vi "Try Parse.vi"(0 "Path Group in":refnum<class "Path Group.lvclass">, 5 "Config Rows":string[][](array[string]), 11 "error in (no error)":errorcluster) -> (4 "Path Group out":refnum<class "Path Group.lvclass">, 6 "Unparsed Rows":string[][](array[string]), 10 "Path Count":i32, 15 "error out":errorcluster)   [LabVIEW 2023, in "RFCalAndFixtureCharact.Common.lvlib" / "Path Group.lvclass"]
uses:
  Path Group.lvclass
  Path/Path.lvclass
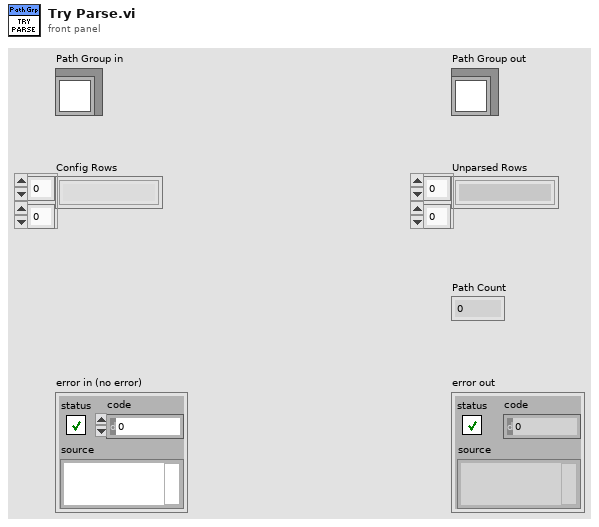
[diagram p1: front panel]
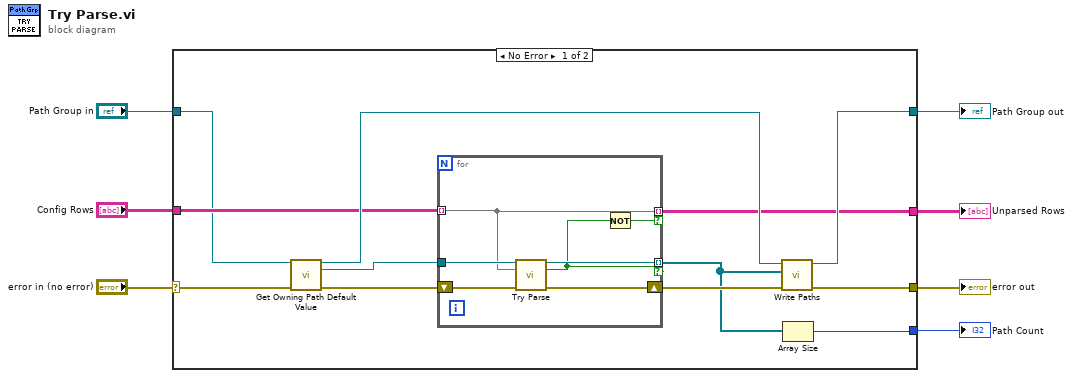
[diagram p0: block diagram]
diagram:
  n1 = case shown="No Error" "error in (no error)" {
    selector: "error in (no error)" -> [w9 w29]
    tunnel: [w18 w29] -> w6
    tunnel: [w17 w28] -> w4
    tunnel: "Path Group in" -> [w8 w28]
    tunnel: [w15 _] -> w3
    tunnel: "Config Rows" -> [w10 w27]
    tunnel: [w11 w27] -> w1
    frame No Error {
      n2 = call-dynamic "Get Owning Path Default Value.vi"("Path Group in"=w8, "error in (no error)"=w9) -> ("Path Group out"=w12:refnum<class "Path Group.lvclass">, "Path"=w13:refnum<class "Path.lvclass">, "error out"=w14:errorcluster)  [unwired: 11 in]
      n3 = for {
        tunnel: w10 -> [w24] mode=indexing
        shift-right: [w21] -> w19
        shift-left: w14 -> [w26]
        tunnel: [w22] -> w16 mode=indexing if=w20
        tunnel: w13 -> [w25]
        tunnel: [w24] -> w11 mode=indexing if=w23
        n4 = call-dynamic "Try Parse.vi"("Path in"=w25, "Config Row"=w24, "error in (no error)"=w26) -> ("Path out"=w22:refnum<class "Path.lvclass">, "Is of type?"=w20:bool, "error out"=w21:errorcluster)  [unwired: 10 in]
        n5 = Not(x=w20) -> (.not. x?=w23:bool)
      }
      n6 = call-dynamic "Write Paths.vi"("error in (no error)"=w19, "Paths"=w16, "Cable Path Group in"=w12) -> ("error out"=w18:errorcluster, "Cable Path Group out"=w17:refnum<class "Path Group.lvclass">)  [unwired: 7 in]
      n7 = Array Size(array=w16) -> (size(s)=w15:i32)
    }
    frame Error {
    }
  }
  "error out" <- w6
  "Path Group out" <- w4
  "Path Count" <- w3
  "Unparsed Rows" <- w1
